vi "Check for Contained Data Type.vi"(6 "LabVIEW Class Qualified Name (\"\")":string, 8 "error in (no error)":errorcluster, 9 "Check Inside Refnums? (F)":bool, 10 "Data Type to Find":T1, 11 "Variant":variant) -> (0 "error out":errorcluster, 3 "Contains Data Type to Find?":bool)   [LabVIEW 2017, in "NI_Data Type.lvlib"]
doc: "Returns TRUE if <B>Variant</B> contains the data type you specify."
uses:
  <vilib>/Utility/Data Type/NI_Data Type.lvlib
  <vilib>/Utility/Data Type/Type Definitions/Data Type.ctl
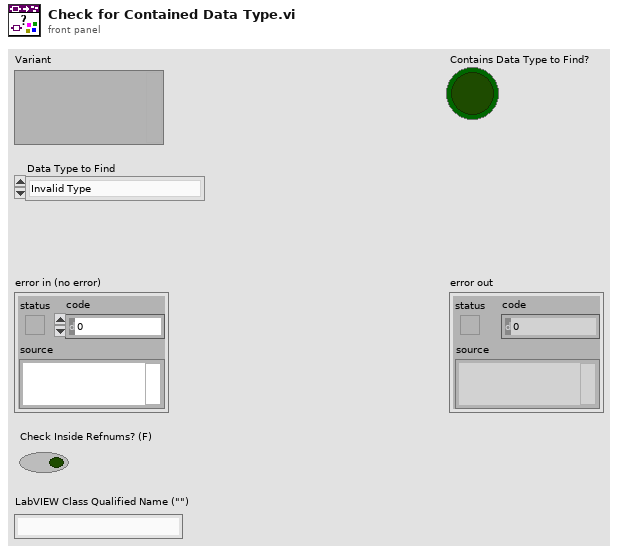
[diagram p1: front panel]
types:
  T1 = typedef "NI_Data Type.lvlib/Data Type.ctl" = enum8{"Invalid Type", "Void", "I8", "I16", "I32", "I64", "U8", "U16", "U32", "U64", "Single Float", "Double Float", "Extended Float", "Single Complex", "Double Complex", "Extended Complex", "Enum U8", "Enum U16", "Enum U32", "Enum U64", "Single Float With Unit", "Double Float With Unit", "Extended Float With Unit", "Single Complex with Unit", "Double Complex with Unit", "Extended Complex with Unit", "Boolean", "String", "Path", "Picture", "Tag", "Array", "Cluster", "Variant", "LV Variant", "Waveform", "Timestamp", "Digital Waveform", "Digital Data", "ExpressData", "Refnum", "External Data", "VI", "Poly VI", "LabVIEW Class Instance", "Fixed Point"}
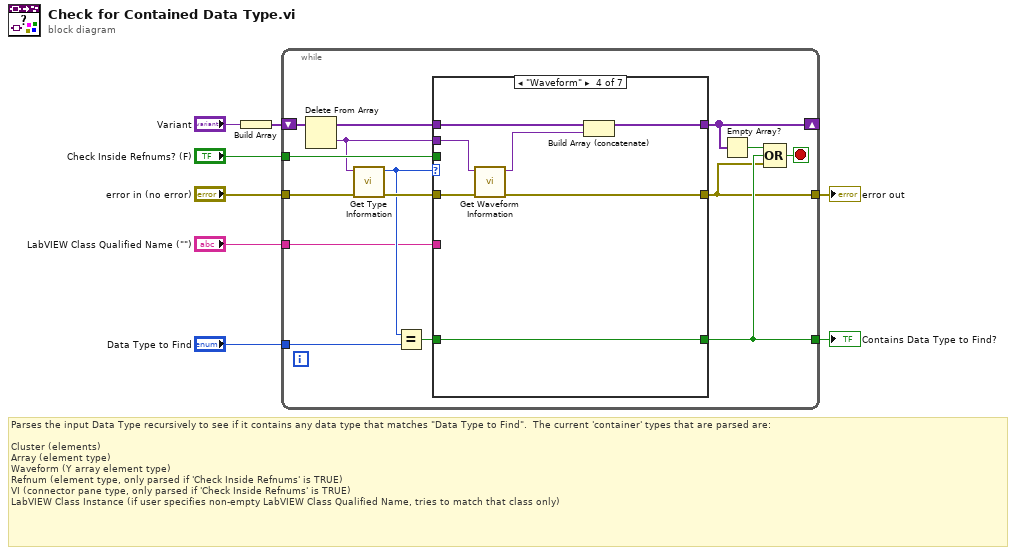
[diagram p0: block diagram]
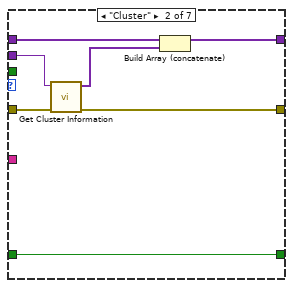
[diagram p3: hidden frame]
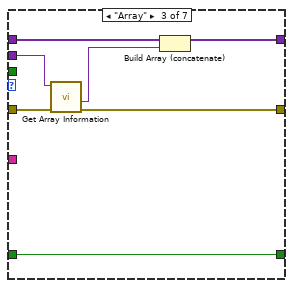
[diagram p4: hidden frame]
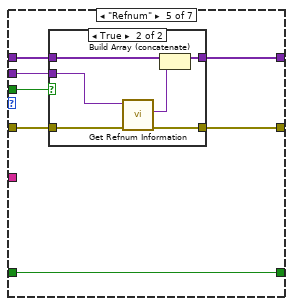
[diagram p5: hidden frame]
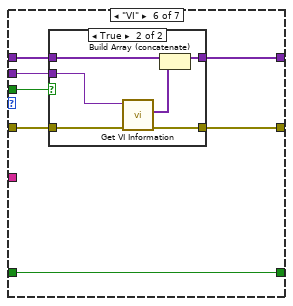
[diagram p7: hidden frame]
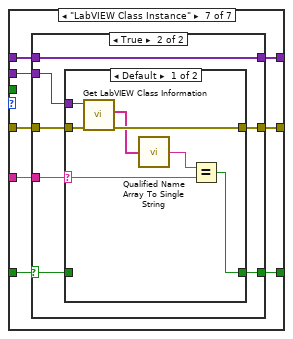
[diagram p9: hidden frame]
diagram:
  # "Parses the input Data Type recursively to see if it contains any data type that matches \"Data Type to Find\".  The current 'container' types that are parsed are:\n\nCluster (elements)\nArray (element type)\nWaveform (Y array element type)\nRefnum (element type, only parsed if 'Check Inside Refnums' is TRUE)\nVI (connector pane type, only parsed if 'Check Inside Refnums' is TRUE)\nLabVIEW Class Instance (if user specifies non-empty LabVIEW Class Qualified Name, tries to match that class only)"
  n1 = Build Array("Variant") -> (w2:variant[])
  n2 = while {
    shift-right: [w19] -> _
    shift-left: w2 -> [w23]
    tunnel: [w11] -> w1
    tunnel: "Data Type to Find" -> [w15]
    tunnel: "Check Inside Refnums? (F)" -> [w14]
    tunnel: "LabVIEW Class Qualified Name (\"\")" -> [w13]
    tunnel: "error in (no error)" -> [w22]
    tunnel: [w10] -> w8
    stop <- w17 stop-if-true
    n3 = Delete From Array(array=w23) -> (deleted portion=w9:variant, array with subset deleted=w20:variant[])  [unwired: 2 in]
    n4 = call <vilib>:"Get Type Information.vi"("error in (no error)"=w22, "Variant"=w9) -> ("error out"=w21:errorcluster, "Type"=w16:T1)  [unwired: 5 in, 3 out]
    n5 = Equal?(x=w16, y=w15) -> (x = y?=w12:bool)
    n6 = case shown="\"Waveform\"" w16 {
      tunnel: w21 -> [w26 w33 w40 w47 w54 w68 w85]
      tunnel: w20 -> [w25 w31 w37 w44 w52 w66 w79]
      tunnel: [w25 w29 w36 w43 w51 w65 w78] -> w19
      tunnel: [w26 w28 w38 w45 w50 w67 w84] -> w10
      tunnel: w9 -> [_ w32 w39 w46 w53 w64 w82]
      tunnel: w14 -> [_ _ _ _ w48 w69 _]
      tunnel: w13 -> [_ _ _ _ _ _ w81]
      tunnel: w12 -> [w24 w27 w34 w41 w49 w63 w80]
      tunnel: [w24 w27 w34 w41 w49 w63 w83] -> w11
      frame Default {
      }
      frame "Cluster" {
        n7 = call <vilib>:"Get Cluster Information.vi"("error in (no error)"=w33, "Variant"=w32) -> ("error out"=w28:errorcluster, "Cluster Elements"=w30:variant[])  [unwired: 8 in]
        n8 = Build Array (concatenate)(w31, w30) -> (w29:variant[])
      }
      frame "Array" {
        n9 = call <vilib>:"Get Array Information.vi"("error in (no error)"=w40, "Variant"=w39) -> ("error out"=w38:errorcluster, "Array Element Data Type"=w35:variant)  [unwired: 6 in, 2 out]
        n10 = Build Array (concatenate)(w37, w35) -> (w36:variant[])
      }
      frame "Waveform" {
        n11 = call <vilib>:"Get Waveform Information.vi"("error in (no error)"=w47, "Variant"=w46) -> ("error out"=w45:errorcluster, "Y Array Type"=w42:variant)  [unwired: 8 in]
        n12 = Build Array (concatenate)(w44, w42) -> (w43:variant[])
      }
      frame "Refnum" {
        n13 = case shown="True" w48 {
          tunnel: w54 -> [w55 w62]
          tunnel: w53 -> [_ w61]
          tunnel: w52 -> [w56 w60]
          tunnel: [w56 w58] -> w51
          tunnel: [w55 w57] -> w50
          frame False {
          }
          frame True {
            n14 = call <vilib>:"Get Refnum Information.vi"("error in (no error)"=w62, "Variant"=w61) -> ("error out"=w57:errorcluster, "Strict Type"=w59:variant)  [unwired: 6 in, 2 out]
            n15 = Build Array (concatenate)(w60, w59) -> (w58:variant[])
          }
        }
      }
      frame "VI" {
        n16 = case shown="True" w69 {
          tunnel: w68 -> [w71 w77]
          tunnel: [w71 w76] -> w67
          tunnel: w66 -> [w70 w74]
          tunnel: [w70 w73] -> w65
          tunnel: w64 -> [_ w75]
          frame False {
          }
          frame True {
            n17 = call <vilib>:"Get VI Information.vi"("error in (no error)"=w77, "Variant"=w75) -> ("error out"=w76:errorcluster, "VI Terminal Types"=w72:variant[])  [unwired: 6 in, 2 out]
            n18 = Build Array (concatenate)(w74, w72) -> (w73:variant[])
          }
        }
      }
      frame "LabVIEW Class Instance" {
        n19 = case shown="True" w80 {
          selector: w80 -> [w86 w90]
          tunnel: w85 -> [w87 w95]
          tunnel: [w87 w94] -> w84
          tunnel: [w86 w93] -> w83
          tunnel: w82 -> [_ w92]
          tunnel: w81 -> [_ w91]
          tunnel: w79 -> [w88 w89]
          tunnel: [w88 w89] -> w78
          frame False {
          }
          frame True {
            n20 = case shown="Default" w91 {
              selector: w91 -> [w99 _]
              tunnel: w90 -> [_ w103]
              tunnel: [w100 w104] -> w94
              tunnel: w95 -> [w102 w104]
              tunnel: [w98 w103] -> w93
              tunnel: w92 -> [w101 _]
              frame Default {
                n21 = call <vilib>:"Get LabVIEW Class Information.vi"("error in (no error)"=w102, "Variant"=w101) -> ("error out"=w100:errorcluster, "Qualified LabVIEW Class Name"=w97:string[])  [unwired: 7 in, 1 out]
                n22 = call <vilib>:"Qualified Name Array To Single String.vi"("Fully Qualified Array"=w97) -> ("Fully Qualified String"=w96:string)
                n23 = Equal?(x=w96, y=w99) -> (x = y?=w98:bool)
              }
              frame "" {
              }
            }
          }
        }
      }
    }
    n24 = Empty Array?(array=w19) -> (empty?=w18:bool)
    n25 = Compound Arithmetic op=OR(w18, w11, w10) -> (w17:bool)
  }
  "Contains Data Type to Find?" <- w1
  "error out" <- w8
